vi "Timing Generator.vi"(6 "primary channel selector":fxp<+,2,0>, 8 "bandwidth":enum16{"20MHz", "40MHz", "80MHz"}(ring), 9 "enable subcarrier counter":bool=TRUE, 10 "format":enum16{"NON_HT_OFDM", "VHT", "NON_HT_DUP_OFDM"}(ring), 11 "OFDM symbol index":u16) -> (2 "Cluster timing":T1={"subcarrier index"=0, "OFDM symbol index"=0, "frequency offset index"=0.0, "OFDM symbol start"=TRUE, "valid"=TRUE})   [LabVIEW 2020]
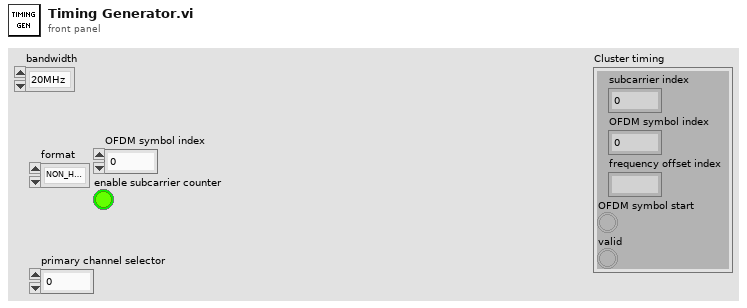
[diagram p1: front panel]
types:
  T1 = cluster{"subcarrier index":u8, "OFDM symbol index":u16, "frequency offset index":fxp<+/-,9,9>, "OFDM symbol start":bool, "valid":bool}
  T2 = cluster{"L-STF-1":bool, "L-STF-2":bool, "L-LTF-1":bool, "L-LTF-2":bool, "L-SIG":bool, "VHT-Data":bool, "VHT-Data Init":bool, "VHT-SIG-B":bool, "VHT-LTF":bool, "VHT-STF":bool, "VHT-SIG A-2":bool, "VHT-SIG A-1":bool, "L-Data":bool, "L-Data Init":bool}
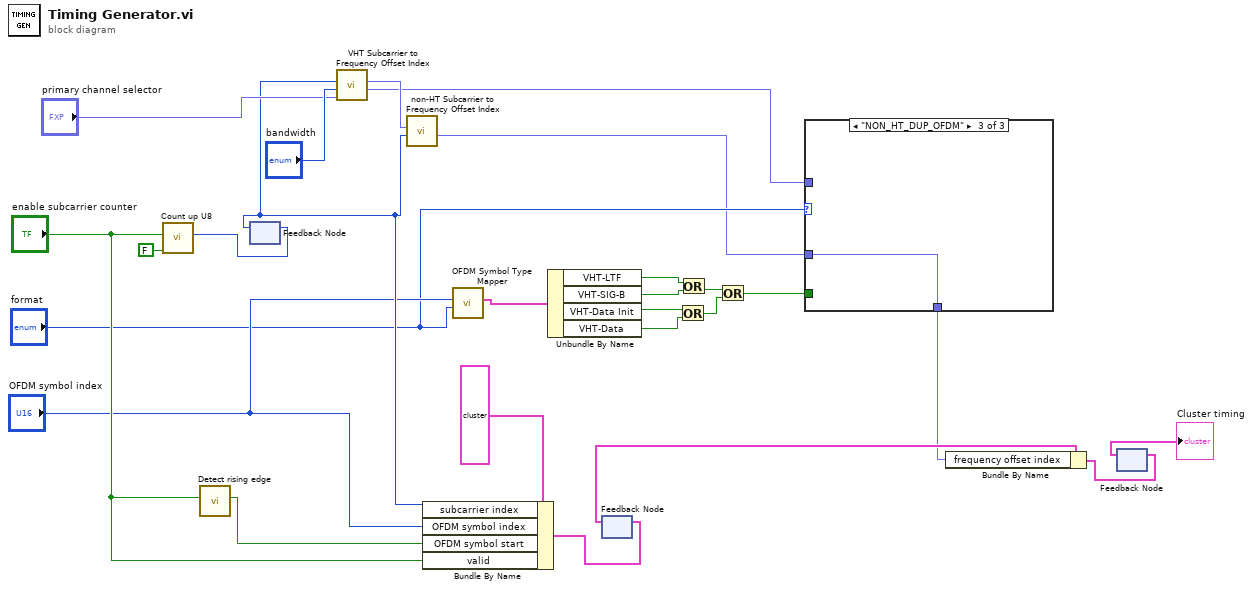
[diagram p0: block diagram]
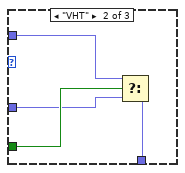
[diagram p3: hidden frame]
diagram:
  n1 = call "Count up U8.vi"("reset"=FALSE, "increment"="enable subcarrier counter") -> ("count out"=w24:u8)  [unwired: 9 in]
  n2 = call "Detect rising edge.vi"("signal"="enable subcarrier counter") -> ("edge detected"=w23:bool)  [unwired: 10 in]
  n3 = feedback-in #1(w24) -> ()
  n4 = feedback #1() -> (w14:u8)  [unwired: 1 in]
  n5 = call "VHT Subcarrier to Frequency Offset Index.vi"("primary channel selector"="primary channel selector", "bandwidth"="bandwidth", "subcarrier index"=w14) -> ("frequency offset index"=w3:fxp<+/-,9,9>, "first non-HT subband"=w15:fxp<+,2,2>)  [unwired: 7 in]
  n6 = call "non-HT Subcarrier to Frequency Offset Index.vi"("subcarrier index"=w14, "primary channel selector"=w15) -> ("frequency offset index"=w2:fxp<+/-,9,9>)  [unwired: 9 in]
  n7 = Bundle By Name(cluster=T1 {"subcarrier index"=0, "OFDM symbol index"=0, "frequency offset index"=0.0, "OFDM symbol start"=TRUE, "valid"=TRUE}, "subcarrier index"=w14, "OFDM symbol index"="OFDM symbol index", "OFDM symbol start"=w23, "valid"="enable subcarrier counter") -> (w21:T1)
  n8 = call "OFDM Symbol Type Mapper.vi"("format"="format", "OFDM symbol index"="OFDM symbol index") -> ("Cluster"=w12:T2)  [unwired: 9 in]
  n9 = Unbundle By Name(w12) -> ("VHT-LTF"=w11:bool, "VHT-SIG-B"=w10:bool, "VHT-Data Init"=w9:bool, "VHT-Data"=w8:bool)
  n10 = feedback #2() -> (w20:T1)  [unwired: 1 in]
  n11 = feedback-in #2(w21) -> ()
  n12 = Or(x=w9, y=w8) -> (x .or. y?=w7:bool)
  n13 = Or(x=w11, y=w10) -> (x .or. y?=w6:bool)
  n14 = Or(x=w6, y=w7) -> (x .or. y?=w4:bool)
  n15 = case shown="\"NON_HT_DUP_OFDM\"" "format" {
    tunnel: w4 -> [_ w31 _]
    tunnel: w3 -> [_ w30 _]
    tunnel: w2 -> [w27 w29 w32]
    tunnel: [w27 w28 w32] -> w1
    frame "NON_HT_OFDM", Default {
    }
    frame "VHT" {
      n16 = Select(t=w30, s=w31, f=w29) -> (s? t:f=w28:fxp<+/-,9,9>)
    }
    frame "NON_HT_DUP_OFDM" {
    }
  }
  n17 = Bundle By Name(cluster=w20, "frequency offset index"=w1) -> (w19:T1)
  n18 = feedback #3() -> (→"Cluster timing":T1)  [unwired: 1 in]
  n19 = feedback-in #3(w19) -> ()
